vi "运维调试_其他.vi"() -> ()   [LabVIEW 2016, in "其他.lvlib"]
uses:
  <vilib>/Utility/miscctls.llb/LVPointTypeDef.ctl
  PLC/PLC.lvlib
  <vilib>/ptbypt/NI_PtbyPt.lvlib
panel:
  out "集成报警信息":string
  out "R115":i16 caption="灯带关闭时间"
  out "R114":i16 caption="灯带开启时间"
  in  "视频监控":bool
  in  "照明":bool
  in  "前门灯带":bool
  in  "侧边灯带":bool
  # "H"
  # "H"
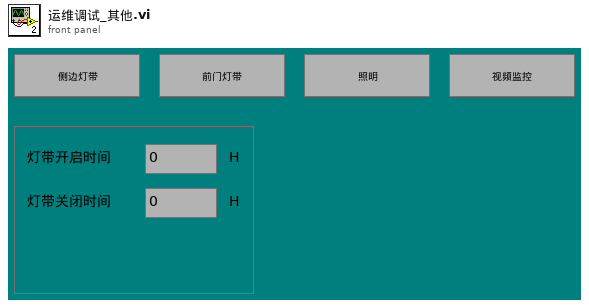
[diagram p1: front panel]
types:
  T1 = cluster{"R100":i16, "R101":i16, "R102":i16, "R103":i16, "R104":i16, "R105":i16, "R106":i16, "R107":i16, "R108":i16, "R109":i16, "R110":i16, "R111":i16, "R112":i16, "R113":i16, "R114":i16, "R115":i16, "R116":i16, "R117":i16, "R118":i16, "R119":i16, "R120":i16, "R121":i16, "R122":i16, "R123":i16}
  T2 = typedef "LVPointTypeDef.ctl" = cluster{"Horizontal":i16, "Vertical":i16}
  T3 = cluster{"命令":string, "data":cluster{"starting address":u16, "coil values":bool[]}}
  T4 = cluster{"命令":string, "数据":cluster{"starting address":u16, "holding register values":u16[]}}
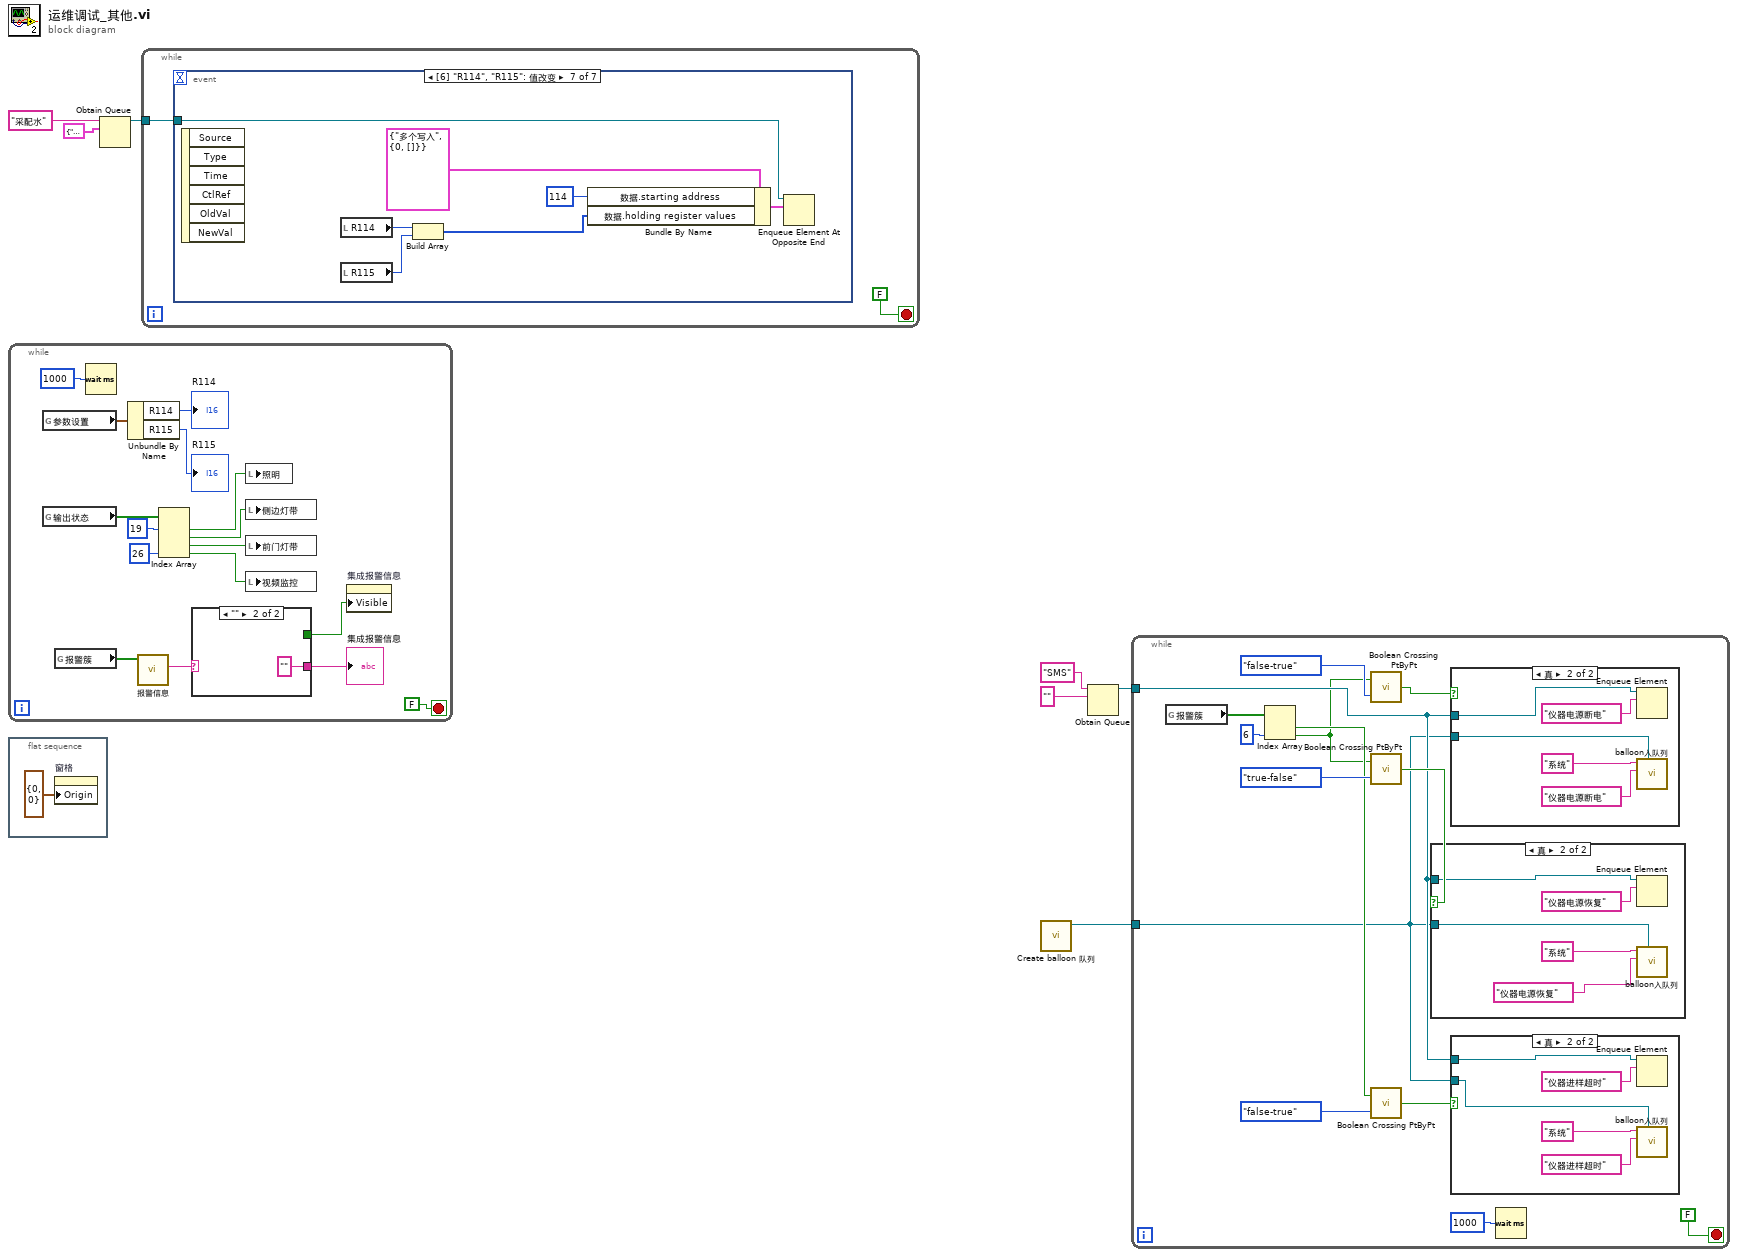
[diagram p0: block diagram]
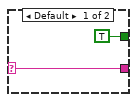
[diagram p5: hidden frame]
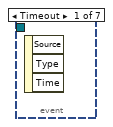
[diagram p6: hidden frame]
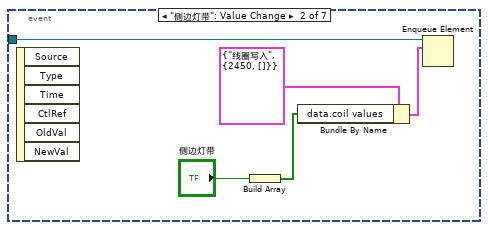
[diagram p7: hidden frame]
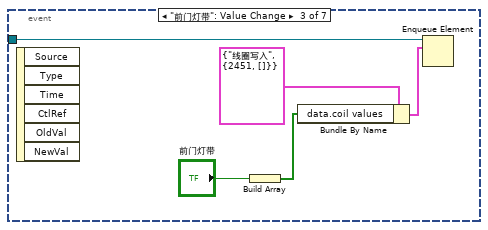
[diagram p8: hidden frame]
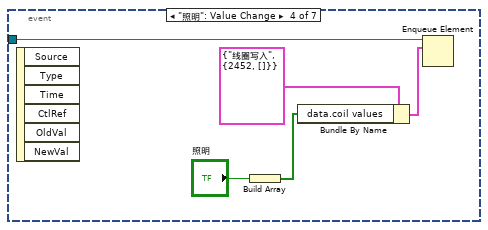
[diagram p9: hidden frame]
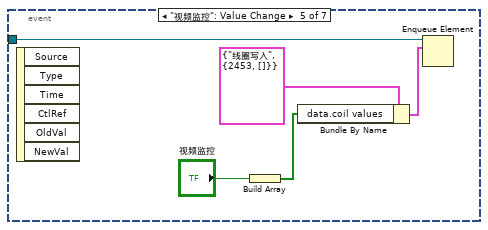
[diagram p10: hidden frame]
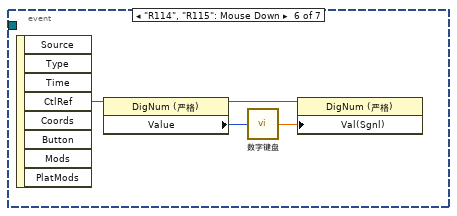
[diagram p11: hidden frame]
diagram:
  n1 = while {
    stop <- FALSE stop-if-true
    n2 = global read "采配水全局变量.vi" "参数设置"() -> (w21:T1)
    n3 = global read "采配水全局变量.vi" "输出状态"() -> (w14:bool[])
    n4 = global read "采配水全局变量.vi" "报警簇"() -> (w15:bool[])
    n5 = Wait (ms)(milliseconds to wait=u32 1000 ("等待时间（毫秒）")) -> ()  [unwired: 1 out]
    n6 = Unbundle By Name(w21) -> ("R114"=→"R114":i16, "R115"=→"R115":i16)
    n7 = call "报警信息.vi"("报警簇"=w15) -> ("系统报警信息"=w18:string)  [unwired: 9 in, 1 out]
    n8 = Index Array(array=w14, index #1=19 ("索引"), index #4=26 ("索引")) -> (element #1=w12:bool, element #2=w11:bool, element #3=w13:bool, element #4=w10:bool)  [unwired: 2 in]
    n9 = case shown="\"\"" w18 {
      selector: w18 -> [w25 _]
      tunnel: [w25 "" ("字符串")] -> w16
      tunnel: [TRUE ("可见") _] -> w17
      frame Default {
      }
      frame "" {
      }
    }
    "集成报警信息" <- w16
    n10 = local write "照明"(w12) -> ()
    n11 = local write "侧边灯带"(w11) -> ()
    n12 = local write "前门灯带"(w13) -> ()
    n13 = local write "视频监控"(w10) -> ()
    n14 = property on="集成报警信息" class="Str"("Visible"=w17) -> ()  [unwired: 2 in, 2 out]
  }
  n15 = flat-sequence {
    frame #0 {
      n16 = property on="窗格" class="Pane"("Origin"=T2 {"Horizontal"=0, "Vertical"=0} ("原点")) -> ()  [unwired: 2 in, 2 out]
    }
  }
  n17 = Obtain Queue(name (unnamed)="采配水" ("名称（未命名）"), element data type=cluster{"命令":string, "数据":variant} {"命令"="", "数据"=variant}) -> (queue out=w5:refnum<queue>)  [unwired: 3 in, 2 out]
  n18 = while {
    tunnel: w5 -> [w28]
    stop <- FALSE stop-if-true
    n19 = event shown="[6] \"R114\", \"R115\": 值改变" {
      selector: _ -> [_ _ _ _ _ _ _]
      dyn-events: _ -> [_ _ _ _ _ _ _]
      timeout: _ -> [_ _ _ _ _ _ _]
      tunnel: w28 -> [_ w31 w37 w42 w47 _ w54]
      event Timeout {
        n20 = event-data() -> ()  [unwired: 1 in, 3 out]
      }
      event "侧边灯带": Value Change {
        n21 = event-data() -> ()  [unwired: 1 in, 6 out]
        n22 = Build Array("侧边灯带") -> (w30:bool[])
        n23 = Bundle By Name(cluster=T3 {"命令"="线圈写入", "data"={"starting address"=2450, "coil values"=[]}} ("元素"), "data.coil values"=w30) -> (w32:T3)
        n24 = Enqueue Element(queue=w31, element=w32) -> ()  [unwired: 2 in, 3 out]
      }
      event "前门灯带": Value Change {
        n25 = event-data() -> ()  [unwired: 1 in, 6 out]
        n26 = Build Array("前门灯带") -> (w36:bool[])
        n27 = Bundle By Name(cluster=T3 {"命令"="线圈写入", "data"={"starting address"=2451, "coil values"=[]}} ("元素"), "data.coil values"=w36) -> (w38:T3)
        n28 = Enqueue Element(queue=w37, element=w38) -> ()  [unwired: 2 in, 3 out]
      }
      event "照明": Value Change {
        n29 = event-data() -> ()  [unwired: 1 in, 6 out]
        n30 = Build Array("照明") -> (w41:bool[])
        n31 = Bundle By Name(cluster=T3 {"命令"="线圈写入", "data"={"starting address"=2452, "coil values"=[]}} ("元素"), "data.coil values"=w41) -> (w43:T3)
        n32 = Enqueue Element(queue=w42, element=w43) -> ()  [unwired: 2 in, 3 out]
      }
      event "视频监控": Value Change {
        n33 = event-data() -> ()  [unwired: 1 in, 6 out]
        n34 = Build Array("视频监控") -> (w46:bool[])
        n35 = Bundle By Name(cluster=T3 {"命令"="线圈写入", "data"={"starting address"=2453, "coil values"=[]}} ("元素"), "data.coil values"=w46) -> (w48:T3)
        n36 = Enqueue Element(queue=w47, element=w48) -> ()  [unwired: 2 in, 3 out]
      }
      event "R114", "R115": Mouse Down {
        n37 = event-data() -> ("CtlRef"=w53:refnum<vi>)  [unwired: 1 in, 7 out]
        n38 = property class="DigNum (严格)"(reference=w53) -> (reference out=w52:refnum<vi>, "Value"=w51:i16)  [unwired: 1 in, 1 out]
        n39 = call "数字键盘.vi"("OldNumber"=w51) -> ("NewNumber"=w50:sgl)
        n40 = property class="DigNum (严格)"(reference=w52, "Val(Sgnl)"=w50) -> ()  [unwired: 1 in, 2 out]
      }
      event "R114", "R115": Value Change {
        n41 = event-data() -> ()  [unwired: 1 in, 6 out]
        n42 = local read "R114"() -> (w59:i16)
        n43 = local read "R115"() -> (w60:i16)
        n44 = Build Array(w59, w60) -> (w55:i16[])
        n45 = Bundle By Name(cluster=T4 {"命令"="多个写入", "数据"={"starting address"=0, "holding register values"=[]}} ("元素"), "数据.starting address"=u16 114, "数据.holding register values"=w55) -> (w56:T4)
        n46 = Enqueue Element At Opposite End(queue=w54, element=w56) -> ()  [unwired: 2 in, 3 out]
      }
    }
  }
  n47 = call "Create balloon 队列.vi"() -> ("队列输出"=w1:refnum<queue>)  [unwired: 11 in]
  n48 = Obtain Queue(name (unnamed)="SMS" ("名称（未命名）"), element data type="" ("名称（未命名）")) -> (queue out=w2:refnum<queue>)  [unwired: 3 in, 2 out]
  n49 = while {
    tunnel: w2 -> [w68]
    tunnel: w1 -> [w61]
    stop <- FALSE stop-if-true
    n50 = global read "采配水全局变量.vi" "报警簇"() -> (w65:bool[])
    n51 = Index Array(array=w65, index #2=6 ("索引")) -> (element #1=w64:bool, element #2=w62:bool)  [unwired: 1 in]
    n52 = call <vilib>:"Boolean Crossing PtByPt.vi"("direction"=enum16{"either", "false-true", "true-false"}."false-true", "input"=w62) -> ("crossing"=w71:bool)  [unwired: 1 in]
    n53 = call <vilib>:"Boolean Crossing PtByPt.vi"("direction"=enum16{"either", "false-true", "true-false"}."true-false", "input"=w62) -> ("crossing"=w69:bool)  [unwired: 1 in]
    n54 = call <vilib>:"Boolean Crossing PtByPt.vi"("direction"=enum16{"either", "false-true", "true-false"}."false-true", "input"=w64) -> ("crossing"=w66:bool)  [unwired: 1 in]
    n55 = case shown="真" w69 {
      tunnel: w68 -> [_ w82]
      tunnel: w61 -> [_ w81]
      frame False {
      }
      frame True {
        n56 = Enqueue Element(queue=w82, element="仪器电源恢复" ("元素")) -> ()  [unwired: 2 in, 3 out]
        n57 = call "balloon入队列.vi"("队列"=w81, "故障信息"="仪器电源恢复" ("元素"), "参数名称"="系统") -> ()  [unwired: 8 in, 1 out]
      }
    }
    n58 = case shown="真" w71 {
      tunnel: w68 -> [_ w89]
      tunnel: w61 -> [_ w87]
      frame False {
      }
      frame True {
        n59 = Enqueue Element(queue=w89, element="仪器电源断电" ("元素")) -> ()  [unwired: 2 in, 3 out]
        n60 = call "balloon入队列.vi"("队列"=w87, "故障信息"="仪器电源断电" ("元素"), "参数名称"="系统") -> ()  [unwired: 8 in, 1 out]
      }
    }
    n61 = case shown="真" w66 {
      tunnel: w68 -> [_ w79]
      tunnel: w61 -> [_ w77]
      frame False {
      }
      frame True {
        n62 = Enqueue Element(queue=w79, element="仪器进样超时" ("元素")) -> ()  [unwired: 2 in, 3 out]
        n63 = call "balloon入队列.vi"("队列"=w77, "故障信息"="仪器进样超时" ("元素"), "参数名称"="系统") -> ()  [unwired: 8 in, 1 out]
      }
    }
    n64 = Wait (ms)(milliseconds to wait=u32 1000 ("等待时间（毫秒）")) -> ()  [unwired: 1 out]
  }
